vi "SetRangeTDC.vi"(7 "Low Range threshold":u16, 8 "error in (no error)":errorcluster, 10 "handle":i32, 11 "VME module Base Address":u32) -> (0 "error out":errorcluster, 2 "VME module Base Address Out":u32, 3 "handle out":i32)   [LabVIEW 2014]
uses:
  Program Files (x86)/CAEN/Comm/labview/CAENComm.lvlib
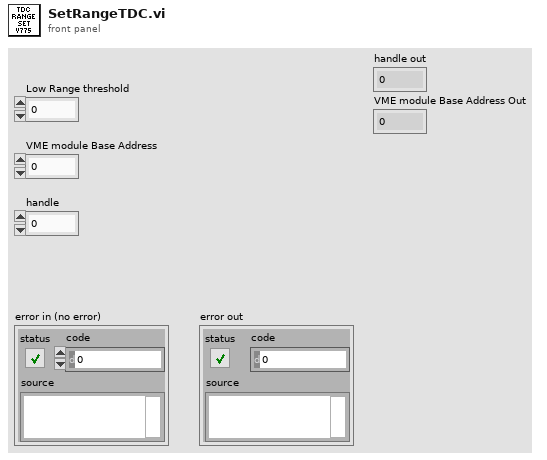
[diagram p1: front panel]
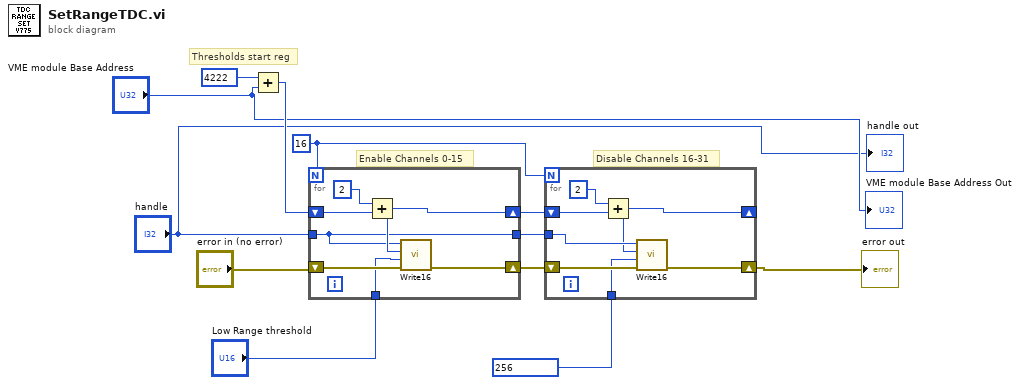
[diagram p0: block diagram]
diagram:
  w4 = 16
  # "Enable Channels 0-15"
  # "Disable Channels 16-31"
  # "Thresholds start reg"
  n1 = Add(x=u32 4222, y="VME module Base Address") -> (x+y=w12:u32)
  n2 = for {
    N: w4 -> [_]
    shift-right: [w14] -> w7
    shift-left: "error in (no error)" -> [w19]
    tunnel: "handle" -> [w13]
    shift-right: [w15] -> w3
    shift-left: w12 -> [w18]
    tunnel: "Low Range threshold" -> [w16]
    tunnel: [w13] -> w6
    n3 = Add(x=u32 2, y=w18) -> (x+y=w15:u32)
    n4 = call "Write16.vi"("error in (no error)"=w19, "Data"=w16, "Address"=w15, "handle"=w13) -> ("error out"=w14:errorcluster)  [unwired: 7 in]
  }
  n5 = for {
    N: w4 -> [_]
    shift-right: [w20] -> w5
    shift-left: w7 -> [w26]
    tunnel: w6 -> [w25]
    shift-right: [w21] -> _
    shift-left: w3 -> [w24]
    tunnel: u16 256 ("Low Range threshold") -> [w22]
    n6 = Add(x=u32 2, y=w24) -> (x+y=w21:u32)
    n7 = call "Write16.vi"("error in (no error)"=w26, "Data"=w22, "Address"=w21, "handle"=w25) -> ("error out"=w20:errorcluster)  [unwired: 7 in]
  }
  "error out" <- w5
  "handle out" <- "handle"
  "VME module Base Address Out" <- "VME module Base Address"
